vi "Flatten Icon.vi"(8 "Error In":errorcluster, 11 "Icon":refnum<class "Icon.lvclass">) -> (0 "Error Out":errorcluster, 3 "String":string)   [LabVIEW 2020]
uses:
  vi.lib/LabVIEW Icon API/lv_icon/Classes/Icon/Icon.lvclass
  vi.lib/LabVIEW Icon API/lv_icon/lv_icon.lvlib
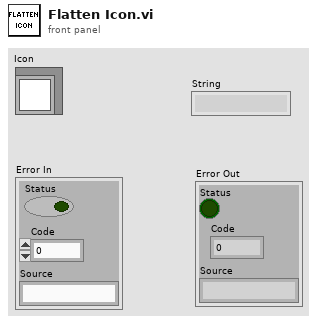
[diagram p1: front panel]
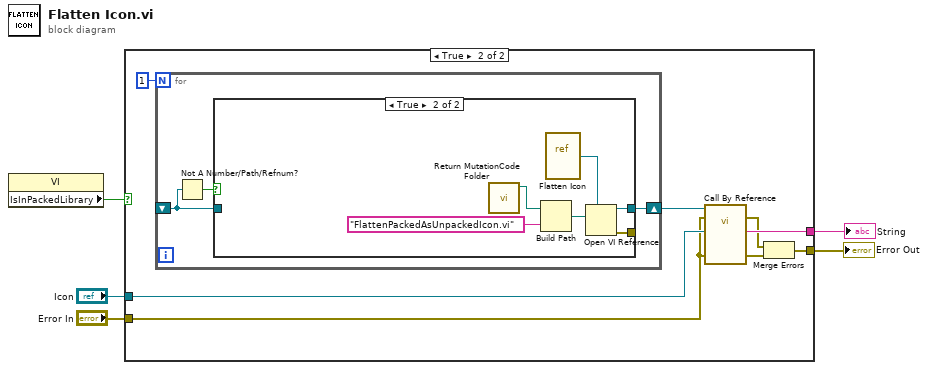
[diagram p0: block diagram]
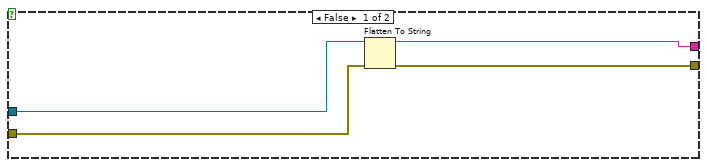
[diagram p2: hidden frame]
diagram:
  n1 = property class="VI"() -> ("IsInPackedLibrary"=w1:bool)  [unwired: 2 in, 2 out]
  n2 = case shown="True" w1 {
    tunnel: [w8 w17] -> w5
    tunnel: "Icon" -> [w6 w16]
    tunnel: "Error In" -> [w7 w15]
    tunnel: [w9 w14] -> w2
    frame False {
      n3 = Flatten To String(anything=w6, error in (no error)=w7) -> (data string=w8:string, error out=w9:errorcluster)  [unwired: 2 in, 1 out]
    }
    frame True {
      n4 = for {
        N: 1 -> [_]
        shift-right: [w18] -> w12
        shift-left: _ -> [w19]
        n5 = Not A Number/Path/Refnum?(number/path/refnum=w19) -> (NaN/Path/Refnum?=w20:bool)
        n6 = case shown="True" w20 {
          tunnel: [w21 w25] -> w18
          tunnel: w19 -> [w21 _]
          tunnel: [_ w22] -> _
          frame False {
          }
          frame True {
            n7 = call "Return MutationCode Folder.vi"() -> ("Base Path Mutation Code"=w24:path)  [unwired: 11 in]
            n8 = Build Path(base path=w24, name or relative path="FlattenPackedAsUnpackedIcon.vi") -> (appended path=w26:path)
            n9 = vi-ref "Flatten Icon.vi"() -> (w23:refnum<vi>)
            n10 = Open VI Reference(type specifier VI Refnum (for type only)=w23, vi path=w26) -> (vi reference=w25:refnum<vi>, error out=w22:errorcluster)  [unwired: 4 in]
          }
        }
      }
      n11 = call-by-ref "?"(reference=w12, error in=w15, "Error In"=w15, "Icon"=w16) -> (error out=w10:errorcluster, "Error Out"=w11:errorcluster, "String"=w17:string)  [unwired: 8 in, 1 out]
      n12 = Merge Errors(w10, w11) -> (w14:errorcluster)
    }
  }
  "String" <- w5
  "Error Out" <- w2
